vi "Mouse Up.vi"(8 "error in (no error)":errorcluster, 10 "Point":T1, 11 "Rectangle in":refnum<class "Rectangle.lvclass">) -> (0 "error out":errorcluster, 3 "Rectangle out":refnum<class "Rectangle.lvclass">)   [LabVIEW 2020, in "Rectangle.lvclass"]
doc: "A method for specifying how a rectangle reacts on a mouse up event"
uses:
  Rectangle.lvclass
  D:/Git/Labview-Libraries/Tools/Drawing Tool Folder/Graphics Object/Graphics Object.lvclass
  D:/Git/Labview-Libraries/Tools/Drawing Tool Folder/Polygon/Polygon.lvclass
  <vilib>/Utility/miscctls.llb/LVPoint32TypeDef.ctl
  Line/Line.lvclass
  Graphics Object/Graphics Object.lvclass
  Polygon/Polygon.lvclass
panel:
  # "expressionflow.com"
  # "Copyright (c) 2008 Tomi Maila. All rights reserved."
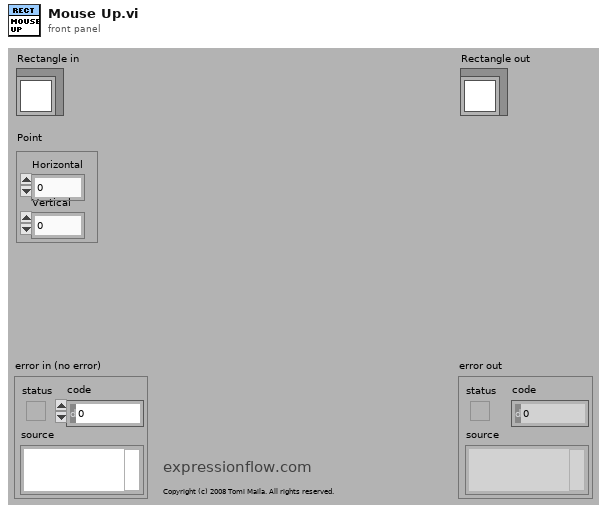
[diagram p1: front panel]
types:
  T1 = typedef "LVPoint32TypeDef.ctl" = cluster{"Horizontal":i32, "Vertical":i32}
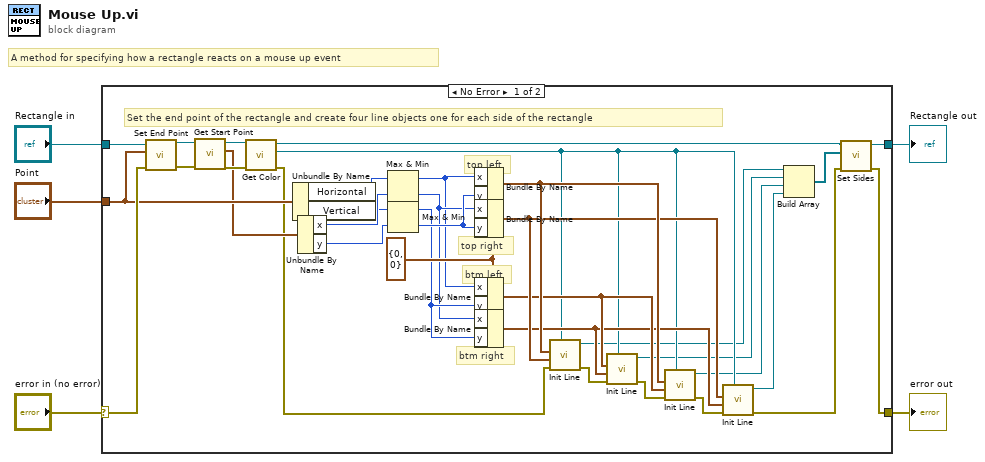
[diagram p0: block diagram]
diagram:
  # "A method for specifying how a rectangle reacts on a mouse up event"
  n1 = case shown="No Error" "error in (no error)" {
    selector: "error in (no error)" -> [w26 w41]
    tunnel: [w10 w41] -> w4
    tunnel: [w14 w42] -> w2
    tunnel: "Rectangle in" -> [w27 w42]
    tunnel: "Point" -> [w21 _]
    frame No Error {
      w39 = cluster{"x":i16, "y":i16} {"x"=0, "y"=0} ("start point")
      # "Set the end point of the rectangle and create four line objects one for each side of the rectangle"
      # "btm right"
      # "btm left"
      # "top right"
      # "top left"
      n2 = call "Set End Point.vi"("error in (no error)"=w26, "end point (0,0)"=w21, "Graphics Object.lvclass in"=w27) -> ("error out"=w22:errorcluster, "Graphics Object.lvclass out"=w25:refnum<class "Rectangle.lvclass">)  [unwired: 7 in]
      n3 = call "Get Start Point.vi"("error in (no error)"=w22, "Graphics Object.lvclass in"=w25) -> ("error out"=w23:errorcluster, "start point"=w20:cluster{"x":i16, "y":i16}, "Graphics Object.lvclass out"=w24:refnum<class "Rectangle.lvclass">)  [unwired: 7 in]
      n4 = call-dynamic "Get Color.vi"("error in (no error)"=w23, "Geometric Object.lvclass in"=w24) -> ("error out"=w15:errorcluster, "Color.lvclass"=w28:refnum<class "Color.lvclass">, "Geometric Object.lvclass out"=w13:refnum<class "Rectangle.lvclass">)  [unwired: 7 in]
      n5 = Unbundle By Name(w21) -> ("Horizontal"=w19:i32, "Vertical"=w17:i32)
      n6 = Unbundle By Name(w20) -> ("x"=w18:i16, "y"=w16:i16)
      n7 = Max & Min(x=w19, y=w18) -> (max(x,y)=w36:i32, min(x,y)=w37:i32)
      n8 = Max & Min(x=w17, y=w16) -> (max(x,y)=w38:i32, min(x,y)=w40:i32)
      n9 = Bundle By Name(cluster=w39, "x"=w36, "y"=w40) -> (w35:cluster{"x":i16, "y":i16})
      n10 = Bundle By Name(cluster=w39, "x"=w37, "y"=w40) -> (w34:cluster{"x":i16, "y":i16})
      n11 = Bundle By Name(cluster=w39, "x"=w36, "y"=w38) -> (w33:cluster{"x":i16, "y":i16})
      n12 = Bundle By Name(cluster=w39, "x"=w37, "y"=w38) -> (w32:cluster{"x":i16, "y":i16})
      n13 = call "Init Line.vi"("Color (RGB black)"=w28, "error in (no error)"=w15, "end point (0,0)"=w34, "start point (0,0)"=w35) -> ("error out"=w29:errorcluster, "Line out"=w9:refnum<class "Line.lvclass">)  [unwired: 6 in]
      n14 = call "Init Line.vi"("Color (RGB black)"=w28, "error in (no error)"=w29, "end point (0,0)"=w32, "start point (0,0)"=w33) -> ("error out"=w30:errorcluster, "Line out"=w8:refnum<class "Line.lvclass">)  [unwired: 6 in]
      n15 = call "Init Line.vi"("Color (RGB black)"=w28, "error in (no error)"=w30, "end point (0,0)"=w33, "start point (0,0)"=w35) -> ("error out"=w31:errorcluster, "Line out"=w7:refnum<class "Line.lvclass">)  [unwired: 6 in]
      n16 = call "Init Line.vi"("Color (RGB black)"=w28, "error in (no error)"=w31, "end point (0,0)"=w32, "start point (0,0)"=w34) -> ("error out"=w11:errorcluster, "Line out"=w6:refnum<class "Line.lvclass">)  [unwired: 6 in]
      n17 = Build Array(w9, w8, w7, w6) -> (w12:refnum<class "Line.lvclass">[])
      n18 = call "Set Sides.vi"("error in (no error)"=w11, "Sides"=w12, "Polygon.lvclass in"=w13) -> ("error out"=w10:errorcluster, "Polygon.lvclass out"=w14:refnum<class "Rectangle.lvclass">)  [unwired: 7 in]
    }
    frame Error {
    }
  }
  "error out" <- w4
  "Rectangle out" <- w2
